vi "BRig_Host__Loop_Producer__UploadClosedLoop__v2.vi"(8 "String":string, 9 "testNewLaserSettings":bool, 10 "input_webdav_status":bool, 11 "session handle":T1) -> ()   [LabVIEW 2014]
uses:
  <vilib>/WebDAVClient/Advanced/SessionHandle.ctl
  <vilib>/WebDAVClient/Advanced/Put File.vi
  <vilib>/WebDAVClient/Advanced/Get File.vi
  <vilib>/WebDAVClient/NI_WebDAV.lvlib
panel:
  out "text 2":string
  out "Get Copy":bool
  out "Sent":bool
  out "text":string
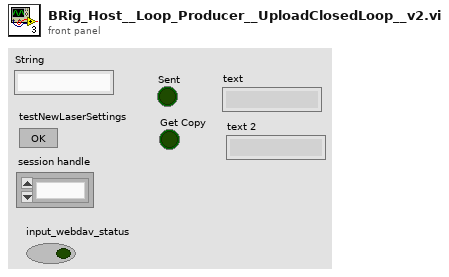
[diagram p1: front panel]
types:
  T1 = typedef "NI_WebDAV.lvlib/SessionHandle.ctl" = refnum<k1>
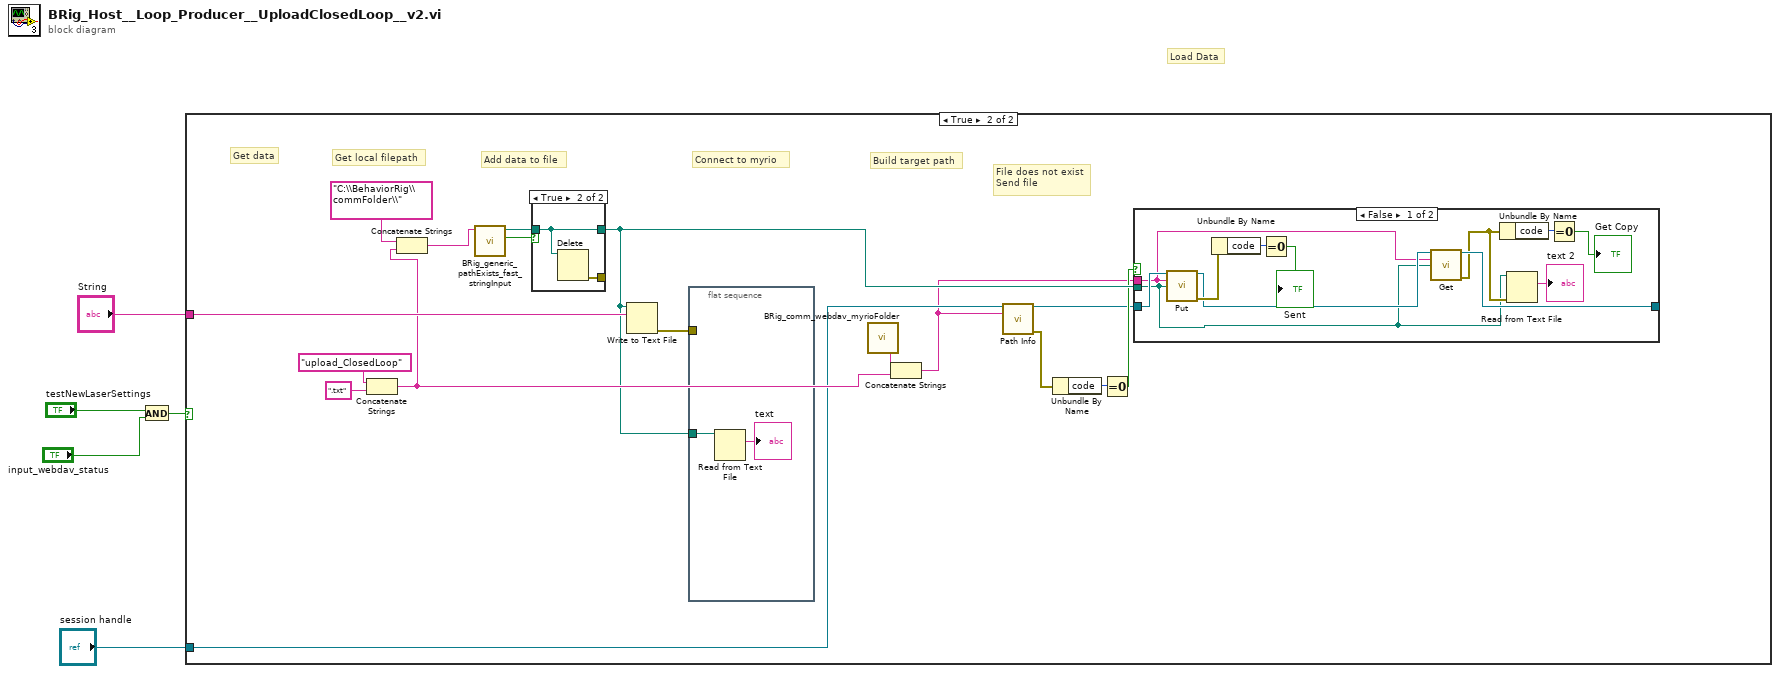
[diagram p0: block diagram]
diagram:
  # "Load Data"
  n1 = And(x="testNewLaserSettings", y="input_webdav_status") -> (x .and. y?=w2:bool)
  n2 = case shown="True" w2 {
    tunnel: "String" -> [_ w20]
    tunnel: "session handle" -> [_ w12]
    frame False {
    }
    frame True {
      # "File does not exist\nSend file"
      # "Build target path"
      # "Connect to myrio"
      # "Add data to file"
      # "Get local filepath"
      # "Get data"
      n3 = Concatenate Strings("upload_ClosedLoop" ("string"), ".txt" ("string")) -> (w15:string)
      n4 = Concatenate Strings("C:\\BehaviorRig\\commFolder\\", w15) -> (w14:string)
      n5 = call "BRig_generic_pathExists_fast_stringInput.vi"("input_filePath"=w14) -> ("output_Iexist"=w22:bool, "output_filePath"=w21:path)  [unwired: 8 in, 1 out]
      n6 = case shown="True" w22 {
        tunnel: w21 -> [w38 w39]
        tunnel: [_ w40] -> _
        tunnel: [w38 w39] -> w13
        frame False {
        }
        frame True {
          n7 = Delete(path (use dialog)=w39) -> (error out=w40:errorcluster)  [unwired: 4 in, 2 out]
        }
      }
      n8 = Write to Text File(file (use dialog)=w13, text=w20) -> (error out=w19:errorcluster)  [unwired: 2 in, 2 out]
      n9 = flat-sequence {
        tunnel: w19 -> [_]
        tunnel: w13 -> [w37]
        frame #0 {
          n10 = Read from Text File(file (use dialog)=w37) -> (text=→"text":string)  [unwired: 3 in, 3 out]
        }
      }
      n11 = call "BRig_comm_webdav_myrioFolder.vi"() -> ("output_myrioFolder"=w11:string)  [unwired: 11 in]
      n12 = Concatenate Strings(w11, w15) -> (w6:string)
      n13 = call <vilib>:"Path Info.vi"("session handle"=w12, "relative uri"=w6) -> ("session handle out"=w7:T1, "error out"=w9:errorcluster)  [unwired: 10 in, 2 out]
      n14 = Unbundle By Name(w9) -> ("code"=w10:i32)
      n15 = Equal To 0?(x=w10) -> (x = 0?=w8:bool)
      n16 = case shown="False" w8 {
        tunnel: w7 -> [w34 w35]
        tunnel: [w29 w35] -> _
        tunnel: w13 -> [w23 _]
        tunnel: w6 -> [w28 _]
        frame False {
          n17 = call-poly <vilib>:"Put.vi"("session handle"=w34, "relative uri"=w28, "local file path"=w23) -> ("session handle out"=w30:T1, "error out"=w32:errorcluster)  [unwired: 10 in, 1 out]
          n18 = Unbundle By Name(w32) -> ("code"=w33:i32)
          n19 = Equal To 0?(x=w33) -> (x = 0?=→"Sent":bool)
          n20 = call-poly <vilib>:"Get.vi"("session handle"=w30, "relative uri"=w28, "local file path"=w23) -> ("session handle out"=w29:T1, "error out"=w24:errorcluster)  [unwired: 10 in, 1 out]
          n21 = Unbundle By Name(w24) -> ("code"=w27:i32)
          n22 = Read from Text File(file (use dialog)=w23, error in=w24) -> (text=→"text 2":string)  [unwired: 2 in, 3 out]
          n23 = Equal To 0?(x=w27) -> (x = 0?=→"Get Copy":bool)
        }
        frame True {
        }
      }
    }
  }
